vi "Initialize IDN.vi"(8 "error in (no error)":errorcluster, 11 "Instrument in":refnum<class "Instrument.lvclass">) -> (0 "error out":errorcluster, 3 "Instrument out":refnum<class "Instrument.lvclass">)   [LabVIEW 2019, in "Instrument.lvclass"]
doc: "Sets the <b>IDN</b> data field:\n- <b>vendor</b> is set by overriding <b>Get SMO Vendor.vi</b>\n- <b>model</b> is set by overriding <b>Get SMO Name.vi</b>\n- <b>serial</b> is set by overriding <b>Get SMO Serial Number.vi</b>\n- <b>firmware</b> refers to the version of your application"
uses:
  Instrument.lvclass
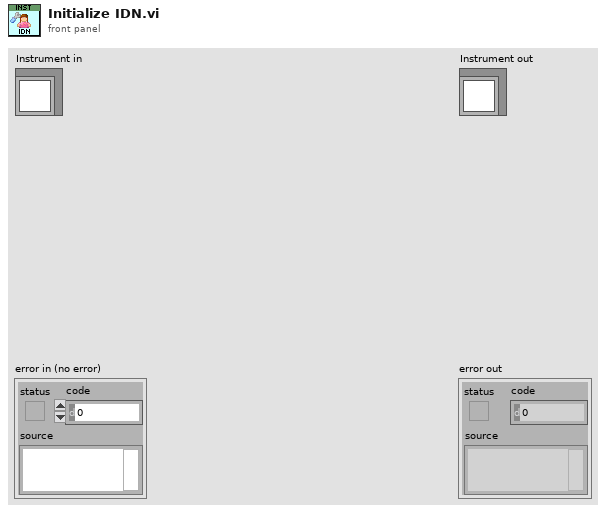
[diagram p1: front panel]
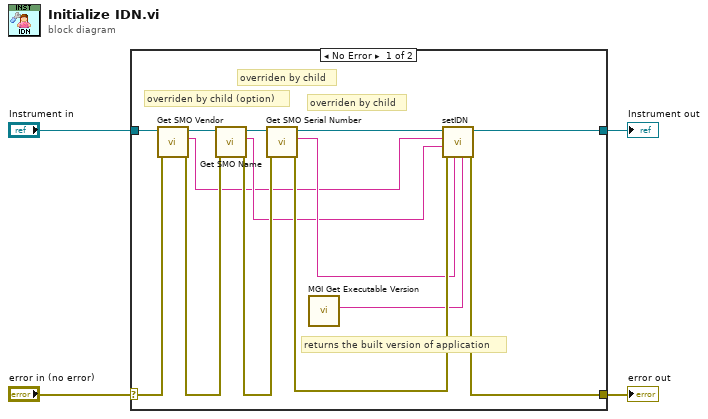
[diagram p0: block diagram]
diagram:
  n1 = case shown="No Error" "error in (no error)" {
    selector: "error in (no error)" -> [w13 w20]
    tunnel: [w9 w20] -> w3
    tunnel: [w16 w19] -> w1
    tunnel: "Instrument in" -> [w15 w19]
    frame No Error {
      # "overriden by child (option)"
      # "returns the built version of application"
      # "overriden by child"
      # "overriden by child"
      n2 = call-dynamic "Get SMO Vendor.vi"("error in (no error)"=w13, "Instrument in"=w15) -> ("error out"=w12:errorcluster, "SMO Vendor"=w5:string, "Instrument out"=w14:refnum<class "Instrument.lvclass">)  [unwired: 7 in]
      n3 = call-dynamic "Get SMO Name.vi"("error in (no error)"=w12, "Instrument in"=w14) -> ("error out"=w18:errorcluster, "SMO Name"=w6:string, "Instrument out"=w11:refnum<class "Instrument.lvclass">)  [unwired: 7 in]
      n4 = call-dynamic "Get SMO Serial Number.vi"("error in (no error)"=w18, "Instrument in"=w11) -> ("error out"=w10:errorcluster, "Serial Number"=w7:string, "Instrument out"=w17:refnum<class "Instrument.lvclass">)  [unwired: 7 in]
      n5 = call <userlib>:"MGI Get Executable Version.vi"() -> ("Version"=w8:string)  [unwired: 7 in]
      n6 = call "setIDN.vi"("Version"=w8, "Serial Number"=w7, "error in (no error)"=w10, "Name"=w6, "Vendor"=w5, "Instrument in"=w17) -> ("error out"=w9:errorcluster, "Instrument out"=w16:refnum<class "Instrument.lvclass">)  [unwired: 4 in]
    }
    frame Error {
    }
  }
  "error out" <- w3
  "Instrument out" <- w1
